vi "Create from SSH.vi"(8 "Error In":errorcluster, 11 "SSH":refnum<class "SSH.lvclass">) -> (0 "Error Out":errorcluster, 3 "Sesssion":refnum<class "Session.lvclass">)   [LabVIEW 2021, in "Field_RnD_Services_LIBSSH2_Toolkit.lvlib" / "Session.lvclass"]
doc: "Create a new Session object from a SSH context."
uses:
  Session.lvclass
  SSH/SSH.lvclass
  Session.lvclass/Session.ctl
  Field_RnD_Services_LIBSSH2_Toolkit.lvlib
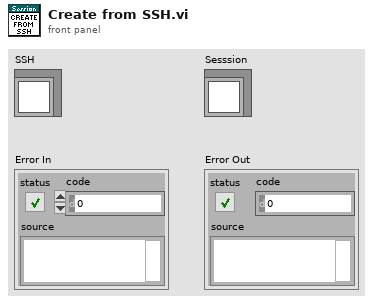
[diagram p1: front panel]
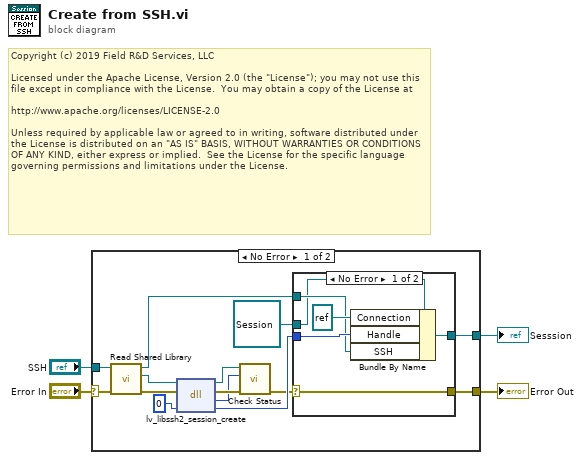
[diagram p0: block diagram]
diagram:
  # "Copyright (c) 2019 Field R&D Services, LLC\n\nLicensed under the Apache License, Version 2.0 (the \"License\"); you may not use this file except in compliance with the License.  You may obtain a copy of the License at\n\nhttp://www.apache.org/licenses/LICENSE-2.0\n\nUnless required by applicable law or agreed to in writing, software distributed under the License is distributed on an \"AS IS\" BASIS, WITHOUT WARRANTIES OR CONDITIONS OF ANY KIND, either express or implied.  See the License for the specific language governing permissions and limitations under the License."
  n1 = case shown="No Error" "Error In" {
    selector: "Error In" -> [w8 w27]
    tunnel: [w11 w27] -> w3
    tunnel: [w18 _] -> w2
    tunnel: "SSH" -> [w10 _]
    frame No Error {
      n2 = call "Read Shared Library.vi"("Error In"=w8, "SSH In"=w10) -> ("Error Out"=w7:errorcluster, "libssh2lv Shared Library"=w9:path, "SSH Out"=w6:refnum<class "SSH.lvclass">)  [unwired: 7 in]
      n3 = dll-call lib="libssh2lv.*" fn="lv_libssh2_session_create"(path in=w9, error in=w7, "handle"=u64 0) -> (path out=w14:path, error out=w15:errorcluster, "status"=w13:i32, "handle"=w16:u64)  [unwired: 1 in]
      n4 = call "Check Status.vi"("Error In"=w15, "Status"=w13, "libssh2lv Shared Library In"=w14) -> ("Error Out"=w12:errorcluster)  [unwired: 7 in, 1 out]
      n5 = case shown="No Error" w12 {
        selector: w12 -> [w21 w26]
        tunnel: [w24 w25] -> w18
        tunnel: w16 -> [w23 _]
        tunnel: [w21 w26] -> w11
        tunnel: w6 -> [w20 _]
        tunnel: refnum<class "Session.lvclass"> refnum ("LabSSH2.lvlib:Session.lvclass") -> [w19 w25]
        frame No Error {
          n6 = Bundle By Name(cluster=w19, "Connection"=refnum<k5> refnum, "Handle"=w23, "SSH"=w20) -> (w24:refnum<class "Session.lvclass">)
        }
        frame Error {
        }
      }
    }
    frame Error {
    }
  }
  "Sesssion" <- w2
  "Error Out" <- w3
